vi "SiosIfmResetManualEnvironment.vi"(0 "Channel":i32(knob) scale=1.0..4.0, 1 "Device Number":i32) -> ()   [LabVIEW 2009]
uses:
  siosifm.dll
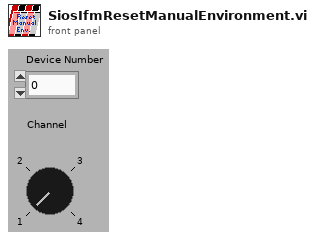
[diagram p1: front panel]
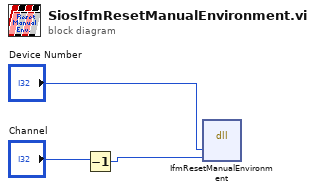
[diagram p0: block diagram]
diagram:
  n1 = Decrement(x="Channel") -> (x-1=w2:i32)
  n2 = dll-call lib="C:/WORK/Artem/RE-10/SIOS_IfmDLL/siosifm.dll" fn="IfmResetManualEnvironment"("devNumber"="Device Number", "channel"=w2) -> ()  [unwired: 6 in, 2 out]
